vi "setSampling.vi"(8 "error in (no error)":errorcluster, 10 "sampling":T1={"Fs"=204789.0, "#s"=15753}, 11 "Instrument.LockinAPI in":refnum<class "Instrument.LockinAPI.lvclass">) -> (0 "error out":errorcluster, 3 "Instrument.LockinAPI out":refnum<class "Instrument.LockinAPI.lvclass">)   [LabVIEW 2019, in "Instrument.LockinAPI.lvclass"]
doc: "API to set sampling configuration (sampling frequency and number of samples)\n\nIf address=\"\", this API reads from localhost\nIf address is remote lockin, you need to add this computer to allowed whitelist on the lockin computer you are trying to access."
uses:
  Instrument.LockinAPI.lvclass
  Typedefs/LockinAPI.Sampling.Sampling--Cluster.ctl
  Typedefs/LockinAPI.Commands--Enum.ctl
  Typedefs/LockinAPI.Sampling.FsMode--enum.ctl
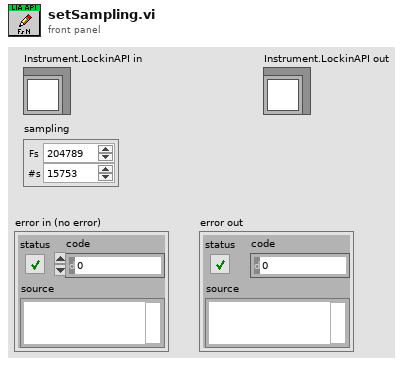
[diagram p1: front panel]
types:
  T1 = typedef "Instrument.LockinAPI.lvclass/LockinAPI.Sampling.Sampling--Cluster.ctl" = cluster{"Fs":dbl, "#s":i32}
  T2 = typedef "Instrument.LockinAPI.lvclass/LockinAPI.Sampling.FsMode--enum.ctl" = enum16{"Manual", "Auto Fs", "Max Fs"}
  T3 = typedef "Instrument.LockinAPI.lvclass/LockinAPI.Commands--Enum.ctl" = enum16{"setAI", "setAO", "setAO_Amplitude", "setAO_DC", "setAO_Frequency", "setAO_Phase", "setAO_Function", "setREF", "setREF_Frequency", "setREF_Phase", "setREF_TC", "setREF_Roll-Off", "setDAQ", "setSampling", "setOffset", "setState", "getState", "getAO", "getAI", "getResults", "getSampling", "getAOconfig", "getREFconfig", "setInputGain", "setOutputGain", "getInputGain", "getOutputGain", "setSamplingFsMode", "getSamplingFsMode", "setSweep", "setSweep_Time", "setSweep_Table", "getStatus", "getSweepResults", "getSweepWaveforms", "startSweep", "stopSweep"}
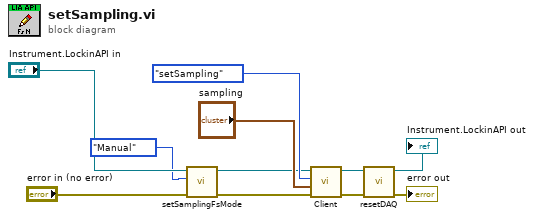
[diagram p0: block diagram]
diagram:
  n1 = call-dynamic "setSamplingFsMode.vi"("error in (no error)"="error in (no error)", "Fs Mode"=LockinAPI.Sampling.FsMode--enum."Manual", "Instrument.LockinAPI in"="Instrument.LockinAPI in") -> ("error out"=w7:errorcluster, "Instrument.LockinAPI out"=w6:refnum<class "Instrument.LockinAPI.lvclass">)  [unwired: 7 in]
  n2 = call-dynamic "Client.vi"("error in (no error)"=w7, "Data in"="sampling", "Command in"=LockinAPI.Commands--Enum."setSampling" ("Command"), "Instrument in"=w6) -> ("error out"=w2:errorcluster, "Instrument out"=w5:refnum<class "Instrument.LockinAPI.lvclass">)  [unwired: 4 in, 2 out]
  n3 = call-dynamic "resetDAQ.vi"("error in (no error)"=w2, "Instrument.LockinAPI in"=w5) -> ("error out"=→"error out":errorcluster, "Instrument.LockinAPI out"=→"Instrument.LockinAPI out":refnum<class "Instrument.LockinAPI.lvclass">)  [unwired: 8 in]
